vi "LUT_InitialScore.vi"() -> (0 "Init Data Out":fxp<+,4,4>[](array[numeric]))   [LabVIEW 2018]
panel:
  out "1/4":i32
  out "number of columns":i32
  out "number of rows":i32
  out "Original":picture
  out "Quotient":i32
  out "Remainder (Must be 0)":i32
  out "TotalPixels":i32
  out "Init Data Out size":i32
  # "For Initialization VI requirements and help, please read directions located on Block Diagram."
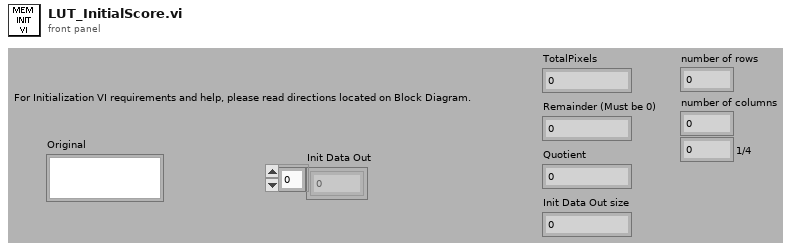
[diagram p1: front panel]
types:
  T1 = typedef "imagedata.ctl" = cluster{"image type":i32, "image depth":i32, "image":u8[], "mask":u8[], "colors":u32[], "Rectangle":cluster{"left":i16, "top":i16, "right":i16, "bottom":i16}}
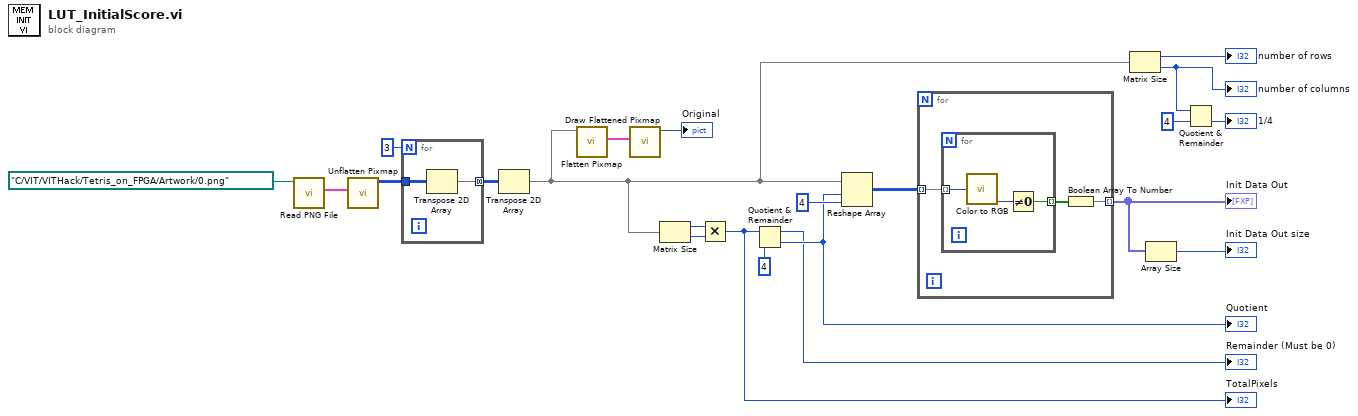
[diagram p0: block diagram]
diagram:
  n1 = call <vilib>:"Read PNG File.vi"("path to PNG file"=path "C:/VIT/VITHack/Tetris_on_FPGA/Artwork/0.png") -> ("image data"=w1:T1)  [unwired: 8 in, 2 out]
  n2 = call <vilib>:"Unflatten Pixmap.vi"("image data"=w1) -> ("24-bit pixmap"=w2:u32[][])  [unwired: 4 in, 6 out]
  n3 = for {
    N: 3 -> [_]
    tunnel: [w24] -> w6 mode=concatenating
    tunnel: w2 -> [w23]
    n4 = Transpose 2D Array(2D array=w23) -> (transposed array=w24:u32[][])
  }
  n5 = Transpose 2D Array(2D array=w6) -> (transposed array=w4:u32[][])
  n6 = call <vilib>:"Flatten Pixmap.vi"("24-bit pixmap"=w4) -> ("image data"=w8:T1)  [unwired: 10 in]
  n7 = call <vilib>:"Draw Flattened Pixmap.vi"("image data"=w8) -> ("new picture"=→"Original":picture)  [unwired: 8 in]
  n8 = Matrix Size(0:w4) -> (1:w16:i32, 2:w15:i32)
  n9 = Multiply(x=w16, y=w15) -> (x*y=w21:i32)
  "TotalPixels" <- w21
  n10 = Quotient & Remainder(x=w21, y=4) -> (x-y*floor(x/y)=→"Remainder (Must be 0)":i32, floor(x/y)=w19:i32)
  "Quotient" <- w19
  n11 = Reshape Array(w4, w19, 4 ("dimension size")) -> (w13:u32[][])
  n12 = for {
    tunnel: w13 -> [w27] mode=indexing
    tunnel: [w26] -> w14 mode=indexing
    n13 = for {
      tunnel: w27 -> [w30] mode=indexing
      tunnel: [w28] -> w25 mode=indexing
      n14 = call <vilib>:"Color to RGB.vi"("Color"=w30) -> ("B"=w29:u8)  [unwired: 3 out]
      n15 = Not Equal To 0?(x=w29) -> (x != 0?=w28:bool)
    }
    n16 = Boolean Array To Number(Boolean array=w25) -> (number=w26:fxp<+,4,4>)
  }
  "Init Data Out" <- w14
  n17 = Matrix Size(0:w4) -> (1:→"number of rows":i32, 2:w11:i32)
  "number of columns" <- w11
  n18 = Array Size(array=w14) -> (size(s)=→"Init Data Out size":i32)
  n19 = Quotient & Remainder(x=w11, y=4) -> (floor(x/y)=→"1/4":i32)  [unwired: 1 out]
